vi "Drive Axis Modifications.vi"(1 "Driver JoyStick Info":T2) -> (0 "Driver JoyStick Info Out":T2)   [LabVIEW 2012]
uses:
  <vilib>/Rock Robotics/WPI/Solenoid/WPI_SolenoidValue.ctl
  Or David (Drive Global Data).vi
panel:
  # "X"
  # "Y"
  # "X"
  # "Y"
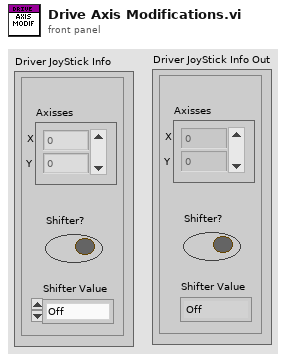
[diagram p1: front panel]
types:
  T1 = typedef "WPI_SolenoidValue.ctl" = enum16{"Off", "On", "Forward", "Reverse"}
  T2 = cluster{"Shifter?":bool, "Axisses":dbl[], "Shifter Value":T1}
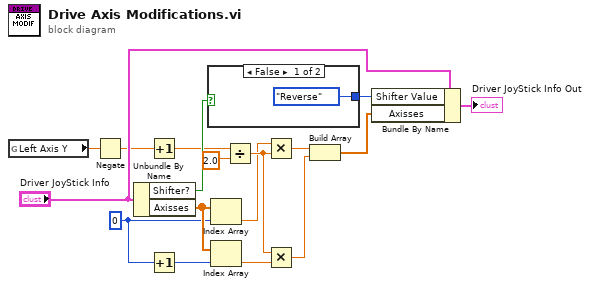
[diagram p0: block diagram]
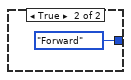
[diagram p2: hidden frame]
diagram:
  w12 = 0 ("index")
  n1 = global read "Or David (Drive Global Data).vi" "Left Axis Y"() -> (w9:dbl)
  n2 = Negate(x=w9) -> (-x=w8:dbl)
  n3 = Unbundle By Name("Driver JoyStick Info") -> ("Shifter?"=w11:bool, "Axisses"=w17:dbl[])
  n4 = Increment(x=w8) -> (x+1=w7:dbl)
  n5 = Increment(x=w12) -> (x+1=w13:i32)
  n6 = case shown="False" w11 {
    tunnel: [WPI_SolenoidValue."Reverse" ("Value") WPI_SolenoidValue."Forward" ("Value")] -> w14
    frame False {
    }
    frame True {
    }
  }
  n7 = Index Array(array=w17, index=w12) -> (element=w3:dbl)
  n8 = Index Array(array=w17, index=w13) -> (element=w2:dbl)
  n9 = Divide(x=w7, y=2.0) -> (x/y=w5:dbl)
  n10 = Multiply(x=w3, y=w5) -> (x*y=w4:dbl)
  n11 = Multiply(x=w5, y=w2) -> (x*y=w1:dbl)
  n12 = Build Array(w4, w1) -> (w10:dbl[])
  n13 = Bundle By Name(cluster="Driver JoyStick Info", "Shifter Value"=w14, "Axisses"=w10) -> (→"Driver JoyStick Info Out":T2)
